vi "Redefine Master.vi"(8 "error in (no error)":errorcluster, 11 "MB_TCP in":refnum<class "MB_TCP.lvclass">) -> (0 "error out":errorcluster, 3 "MB_TCP out":refnum<class "MB_TCP.lvclass">)   [LabVIEW 2021, in "MB_TCP.lvclass"]
uses:
  MB_TCP.lvclass
  NI_modbus_upd/TCP/tcp timeouts.ctl
  MB_TCP.lvclass/MB_TCP.ctl
  NI_modbus_upd/TCP/TCP.lvclass/TCP.ctl
  NI_modbus_upd/TCP/TCP.lvclass
  ICPCON Param/ICPCON_Param.lvlib
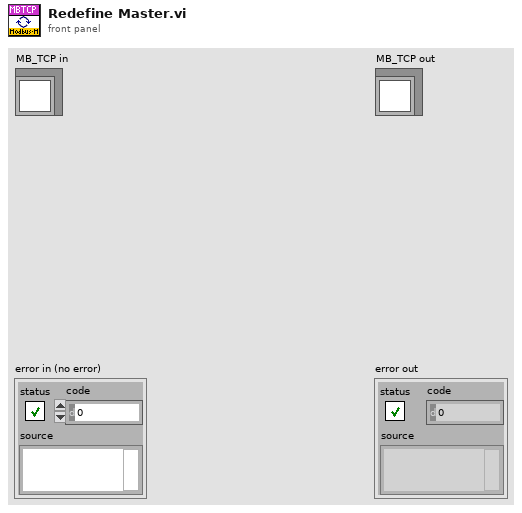
[diagram p1: front panel]
types:
  T1 = typedef "TCP.lvclass/tcp timeouts.ctl" = cluster{"connect timeout":i32, "write timeout":i32, "read timeout":i32}
  T2 = typedef "ICPCON_Param.lvlib/ICPCON Param.ctl" = cluster{"IP addr":refnum<data-value>, "MVIName":refnum<data-value>, "timeouts":refnum<data-value>, "modified":refnum<data-value>}
  T3 = cluster{"Remote IP Address":string, "Remote Port":u16}
  T4 = typedef "ICPCON_Param.lvlib/Eth timeouts.ctl" = cluster{"conn_timeout":i32, "reconn_timeout":i32, "N attempt max":i32, "t_reset_TTL":i32, "write_timeout":i32, "read_timeout":i32, "period":i32}
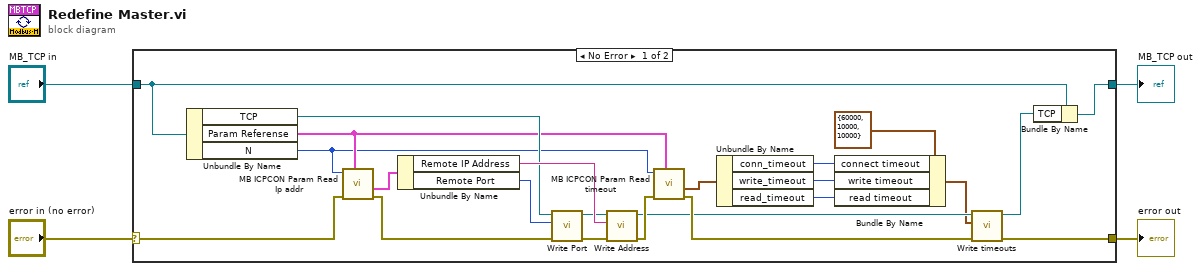
[diagram p0: block diagram]
diagram:
  n1 = case shown="No Error" "error in (no error)" {
    selector: "error in (no error)" -> [w8 w28]
    tunnel: [w7 w28] -> w1
    tunnel: [w5 w29] -> w2
    tunnel: "MB_TCP in" -> [w6 w29]
    frame No Error {
      n2 = Unbundle By Name(w6) -> ("TCP"=w21:refnum<class "TCP.lvclass">, "Param Referense"=w20:T2, "N"=w18:i32)
      n3 = call "MB ICPCON Param Read Ip addr.vi"("Param Reference"=w20, "error in (no error)"=w8, "N"=w18) -> ("error out"=w22:errorcluster, "IP address"=w27:T3)  [unwired: 7 in]
      n4 = Unbundle By Name(w27) -> ("Remote IP Address"=w26:string, "Remote Port"=w25:u16)
      n5 = call "Write Port.vi"("error in (no error)"=w22, "port"=w25, "TCP in"=w21) -> ("error out"=w23:errorcluster, "TCP out"=w24:refnum<class "TCP.lvclass">)  [unwired: 7 in]
      n6 = call "Write Address.vi"("error in (no error)"=w23, "address"=w26, "TCP in"=w24) -> ("error out"=w19:errorcluster, "TCP out"=w11:refnum<class "TCP.lvclass">)  [unwired: 7 in]
      n7 = call "MB ICPCON Param Read timeout.vi"("Param Reference"=w20, "error in (no error)"=w19, "N"=w18) -> ("error out"=w17:errorcluster, "timeout"=w16:T4)  [unwired: 7 in]
      n8 = Unbundle By Name(w16) -> ("conn_timeout"=w15:i32, "write_timeout"=w13:i32, "read_timeout"=w12:i32)
      n9 = Bundle By Name(cluster=T1 {"connect timeout"=60000, "write timeout"=10000, "read timeout"=10000} ("timeouts"), "connect timeout"=w15, "write timeout"=w13, "read timeout"=w12) -> (w10:T1)
      n10 = call "Write timeouts.vi"("error in (no error)"=w17, "timeouts"=w10, "TCP Master in"=w11) -> ("error out"=w7:errorcluster, "TCP Master out"=w9:refnum<class "TCP.lvclass">)  [unwired: 7 in]
      n11 = Bundle By Name(cluster=w6, "TCP"=w9) -> (w5:refnum<class "MB_TCP.lvclass">)
    }
    frame Error {
    }
  }
  "error out" <- w1
  "MB_TCP out" <- w2
